vi "初始化查询数组(子VI).vi"(8 "error in (no error)":errorcluster caption="错误输入（无错误）", 11 "Table输入":refnum<vi>) -> (0 "error out":errorcluster caption="错误输出")   [LabVIEW 2016]
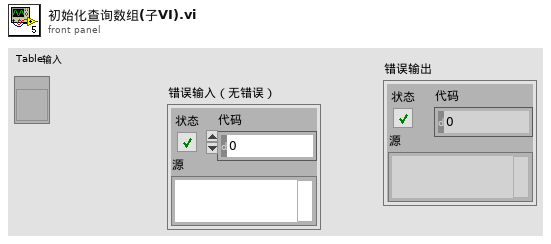
[diagram p1: front panel]
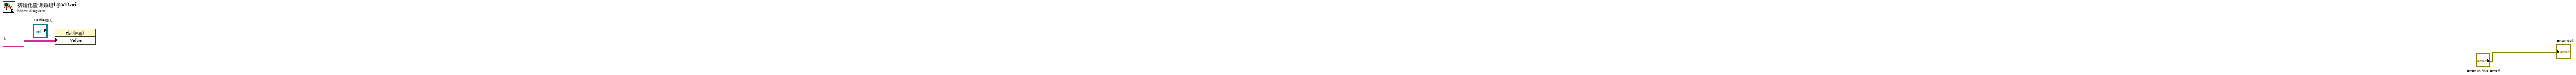
[diagram p0: block diagram]
diagram:
  n1 = property class="Tbl (严格)"(reference="Table输入", "Value"=string[][] []) -> ()  [unwired: 1 in, 2 out]
  "error out" <- "error in (no error)"
